vi "Keep Launcher Alive While Running App.vi"(8 "error in (no error)":errorcluster) -> (0 "error out":errorcluster)   [LabVIEW 2021, in "Architecture.lvlib"]
uses:
  Architecture.lvlib
  Typedefs/FGV Ref. Modules Function.ctl
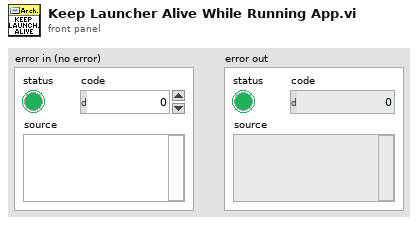
[diagram p1: front panel]
types:
  T1 = typedef "Architecture.lvlib/FGV Ref. Modules Function.ctl" = enum16{"Init ", "Add Module", "Get Module", "Get All", "Add Asynchronous Run Ref", "Dispose"}
  T2 = typedef "Architecture.lvlib/Module References.ctl" = cluster{"ModuleName":T3, "Queue":refnum<queue>, "user event":refnum<user-event>, "VI Refnum":refnum<vi>, "ShowFP":bool, "StatesTracking Enabled":bool}
  T3 = typedef "Configuration.lvlib/Enum_Module_Name.ctl" = enum16{"Configuration", "Error_Handler", "Log", "Database", "Controller", "UI Module", "Sound Manager"}
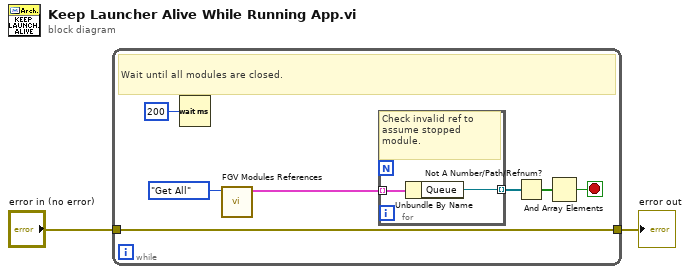
[diagram p0: block diagram]
diagram:
  n1 = while {
    tunnel: "error in (no error)" -> [w3]
    tunnel: [w3] -> w2
    stop <- w9 stop-if-true
    # "Wait until all modules are closed."
    n2 = Wait (ms)(milliseconds to wait=u32 200) -> ()  [unwired: 1 out]
    n3 = call "FGV Modules References.vi"("FGV Ref. Function In"=FGV_Ref._Modules_Function."Get All") -> ("All Modules Refs"=w7:T2[])  [unwired: 7 in, 3 out]
    n4 = for {
      tunnel: w7 -> [w11] mode=indexing
      tunnel: [w10] -> w6 mode=indexing
      # "Check invalid ref to assume stopped module."
      n5 = Unbundle By Name(w11) -> ("Queue"=w10:refnum<queue>)
    }
    n6 = Not A Number/Path/Refnum?(number/path/refnum=w6) -> (NaN/Path/Refnum?=w5:bool[])
    n7 = And Array Elements(Boolean array=w5) -> (logical AND=w9:bool)
  }
  "error out" <- w2
